vi "Wait - Copy.vi"(11 "Time":dbl) -> ()   [LabVIEW 2017]
uses:
  RoutineData.vi
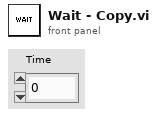
[diagram p1: front panel]
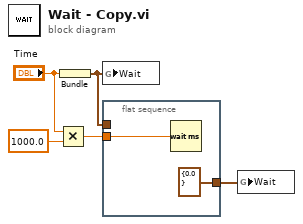
[diagram p0: block diagram]
diagram:
  n1 = Multiply(x="Time", y=1000.0) -> (x*y=w1:dbl)
  n2 = Bundle("Time"="Time") -> (w5:cluster{"Time":dbl})  [unwired: 1 in]
  n3 = global write "RoutineData.vi" "Wait"(w5) -> ()
  n4 = flat-sequence {
    tunnel: w5 -> [_]
    tunnel: [cluster{"Distance":dbl} {"Distance"=0.0} ("output cluster")] -> w4
    tunnel: w1 -> [w6]
    frame #0 {
      n5 = Wait (ms)(milliseconds to wait=w6) -> ()  [unwired: 1 out]
    }
  }
  n6 = global write "RoutineData.vi" "Wait"(w4) -> ()
